vi "WriteDataQvb.vi"(8 "error in (no error)":errorcluster caption="entrée d'erreur (pas d'erreur)", 9 "IndPoint":i32, 10 "DataIn":dbl[](array[numeric]), 11 "Interface en entrée":refnum<class "Interface.lvclass"> caption="DNL_LabVIEW Object in") -> (0 "error out":errorcluster caption="sortie d'erreur", 1 "CrvIndex":i32, 2 "CurCrvPointInd":i32, 3 "Interface en sortie":refnum<class "Interface.lvclass"> caption="DNL_LabVIEW Object out", 4 "ScanTableSize":i32[](array[numeric]))   [LabVIEW 2019, in "Interface.lvclass"]
uses:
  Interface.lvclass
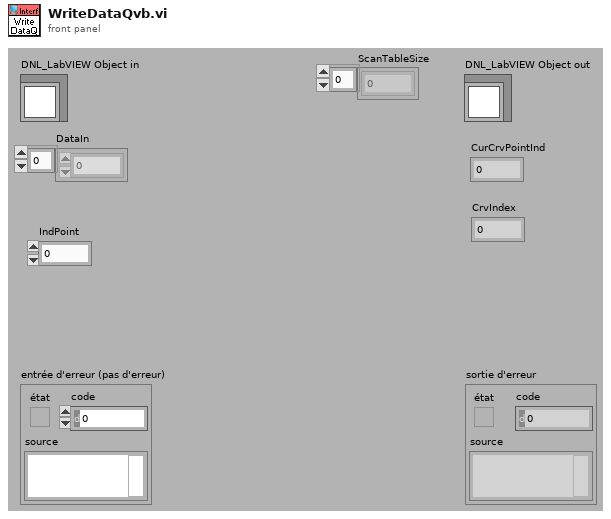
[diagram p1: front panel]
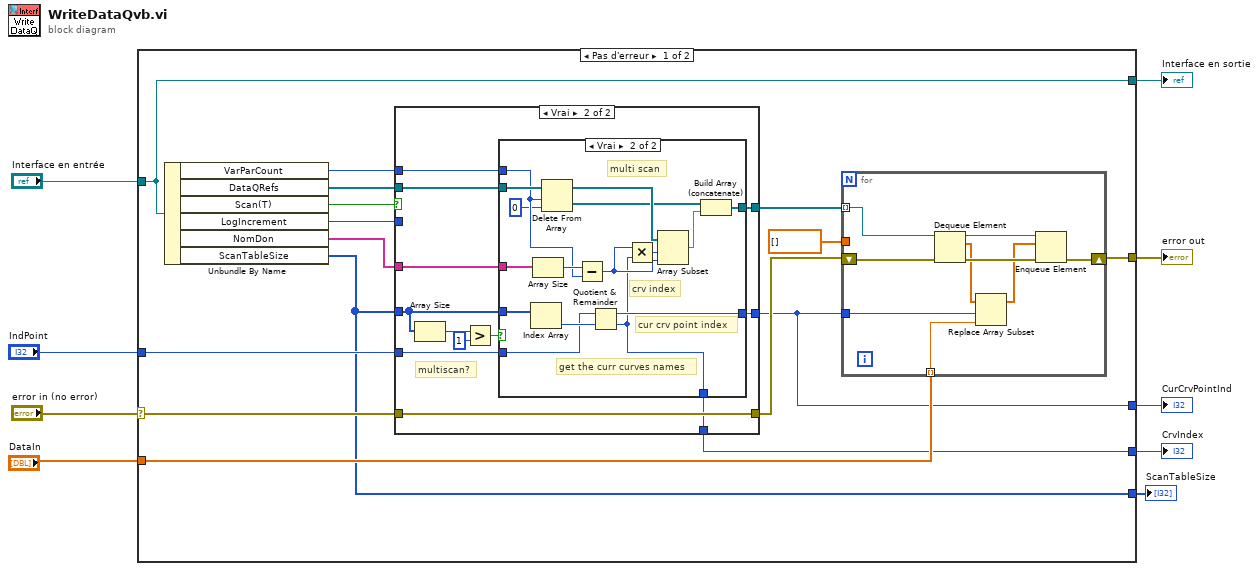
[diagram p0: block diagram]
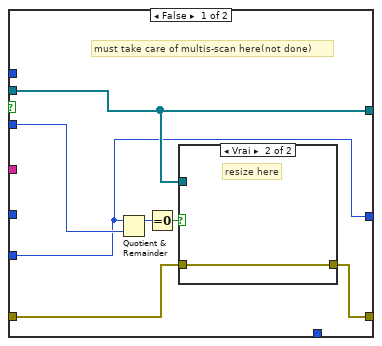
[diagram p2: hidden frame]
diagram:
  n1 = case shown="Pas d'erreur" "error in (no error)" {
    selector: "error in (no error)" -> [w14 w75]
    tunnel: [w25 w75] -> w8
    tunnel: [w20 w74] -> w6
    tunnel: "Interface en entrée" -> [w20 w74]
    tunnel: "DataIn" -> [w23 _]
    tunnel: "IndPoint" -> [w19 _]
    tunnel: [w12 _] -> w3
    tunnel: [w11 _] -> w2
    tunnel: [w10 _] -> w1
    frame No Error {
      n2 = Unbundle By Name(w20) -> ("VarParCount"=w13:i32, "DataQRefs"=w15:refnum<queue>[], "Scan(T)"=w17:bool, "LogIncrement"=w22:i32, "NomDon"=w18:string[], "ScanTableSize"=w10:i32[])
      n3 = case shown="Vrai" w17 {
        tunnel: w22 -> [w30 _]
        tunnel: w19 -> [w26 w45]
        tunnel: w14 -> [w29 w46]
        tunnel: [w28 w46] -> w21
        tunnel: w10 -> [_ w42]
        tunnel: w18 -> [_ w44]
        tunnel: w15 -> [w27 w38]
        tunnel: [w27 w43] -> w16
        tunnel: w13 -> [_ w37]
        tunnel: [w26 w36] -> w12
        tunnel: [_ w35] -> w11
        frame False {
          # "must take care of multis-scan here(not done)"
          n4 = Quotient & Remainder(x=w26, y=w30) -> (x-y*floor(x/y)=w32:i32)  [unwired: 1 out]
          n5 = Equal To 0?(x=w32) -> (x = 0?=w31:bool)
          n6 = case shown="Vrai" w31 {
            tunnel: w27 -> [_ _]
            tunnel: w29 -> [w33 w34]
            tunnel: [w33 w34] -> w28
            frame False {
            }
            frame True {
              # "resize here"
            }
          }
        }
        frame True {
          # "multiscan?"
          n7 = Array Size(array=w42) -> (size(s)=w41:i32)
          n8 = Greater?(x=w41, y=1) -> (0:w39:bool)
          n9 = case shown="Vrai" w39 {
            tunnel: w45 -> [w47 w63]
            tunnel: w44 -> [_ w62]
            tunnel: w38 -> [w48 w60]
            tunnel: [w48 w59] -> w43
            tunnel: w42 -> [_ w61]
            tunnel: w37 -> [_ w55]
            tunnel: [w47 w50] -> w36
            tunnel: [_ w49] -> w35
            frame False {
              # "single scan"
            }
            frame True {
              # "crv index"
              # "cur crv point index"
              # "multi scan"
              # "get the curr curves names"
              n10 = Index Array(array=w61) -> (element=w64:i32)  [unwired: 1 in]
              n11 = Array Size(array=w62) -> (size(s)=w56:i32)
              n12 = Delete From Array(array=w60, length=w55, index=0 ("indice")) -> (deleted portion=w57:refnum<queue>[], array with subset deleted=w58:refnum<queue>[])
              n13 = Subtract(x=w56, y=w55) -> (x-y=w52:i32)
              n14 = Quotient & Remainder(x=w63, y=w64) -> (x-y*floor(x/y)=w50:i32, floor(x/y)=w49:i32)
              n15 = Multiply(x=w52, y=w49) -> (x*y=w53:i32)
              n16 = Array Subset(array=w58, index=w53, length=w52) -> (w54:refnum<queue>[])
              n17 = Build Array (concatenate)(w57, w54) -> (w59:refnum<queue>[])
            }
          }
        }
      }
      n18 = for {
        shift-right: [w72] -> w25
        shift-left: w21 -> [w65]
        tunnel: w23 -> [w68] mode=indexing
        tunnel: w12 -> [w67]
        tunnel: dbl[] [] ("élément") -> [_]
        tunnel: w16 -> [w66] mode=indexing
        n19 = Dequeue Element(queue=w66, error in (no error)=w65) -> (queue out=w73:refnum<queue>, element=w70:dbl[], error out=w71:errorcluster)  [unwired: 1 in, 1 out]
        n20 = Replace Array Subset(array=w70, new element=w68, index=w67) -> (w69:dbl[])
        n21 = Enqueue Element(queue=w73, element=w69, error in (no error)=w71) -> (error out=w72:errorcluster)  [unwired: 1 in, 2 out]
      }
    }
    frame Error {
    }
  }
  "error out" <- w8
  "Interface en sortie" <- w6
  "CurCrvPointInd" <- w3
  "CrvIndex" <- w2
  "ScanTableSize" <- w1
